vi "Calc - SGCAL.vi"(10 "RhoH20":dbl, 11 "RhoFuel":dbl) -> (3 "SGCAL":dbl)   [LabVIEW 2018, in "Controller (Host).lvlib"]
uses:
  Controller (Host).lvlib
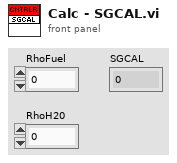
[diagram p1: front panel]
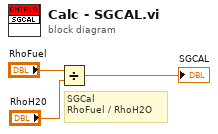
[diagram p0: block diagram]
diagram:
  # "SGCal\nRhoFuel / RhoH2O"
  n1 = Divide(x="RhoFuel", y="RhoH20") -> (x/y=→"SGCAL":dbl)
